vi "_readCmdFromExcel_EEPROM_vna_wmg.vi"(11 "命令类型选择":string(combo)) -> (3 "cmd":string[][](array[string]))   [LabVIEW 2011]
uses:
  <vilib>/Utility/file.llb/Read From Spreadsheet File (string).vi
  <vilib>/Utility/file.llb/Write To Spreadsheet File (string).vi
panel:
  in  "file path (dialog if empty)":path=path "\\\\192.168.20.200\\立讯精密/工程部/电子&测试工程课/临时文件/WMG/HPTS/HPTS_VNA Test System/EEPROM/Commands/Commands1.xls" caption="文件路径 （空时为对话框）"
  out "Loop":i32=5
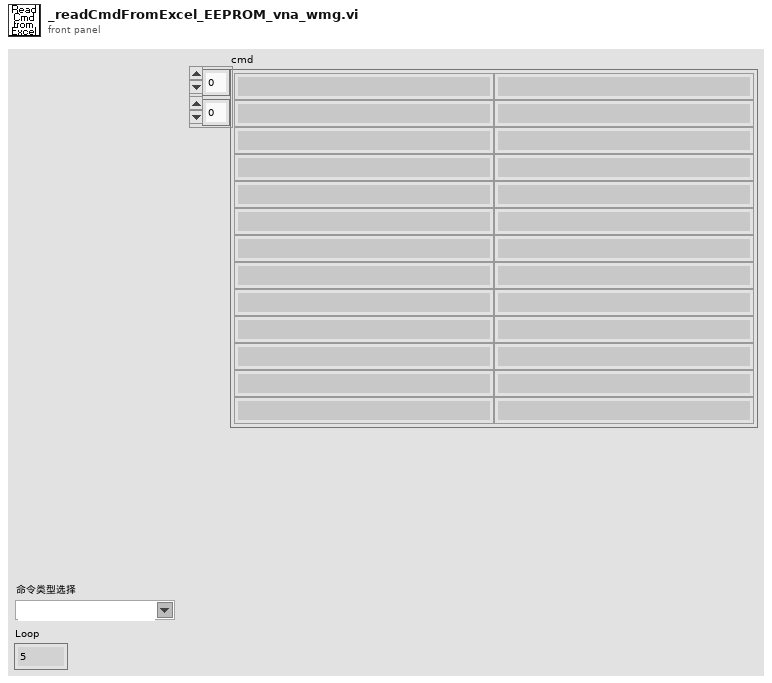
[diagram p1: front panel]
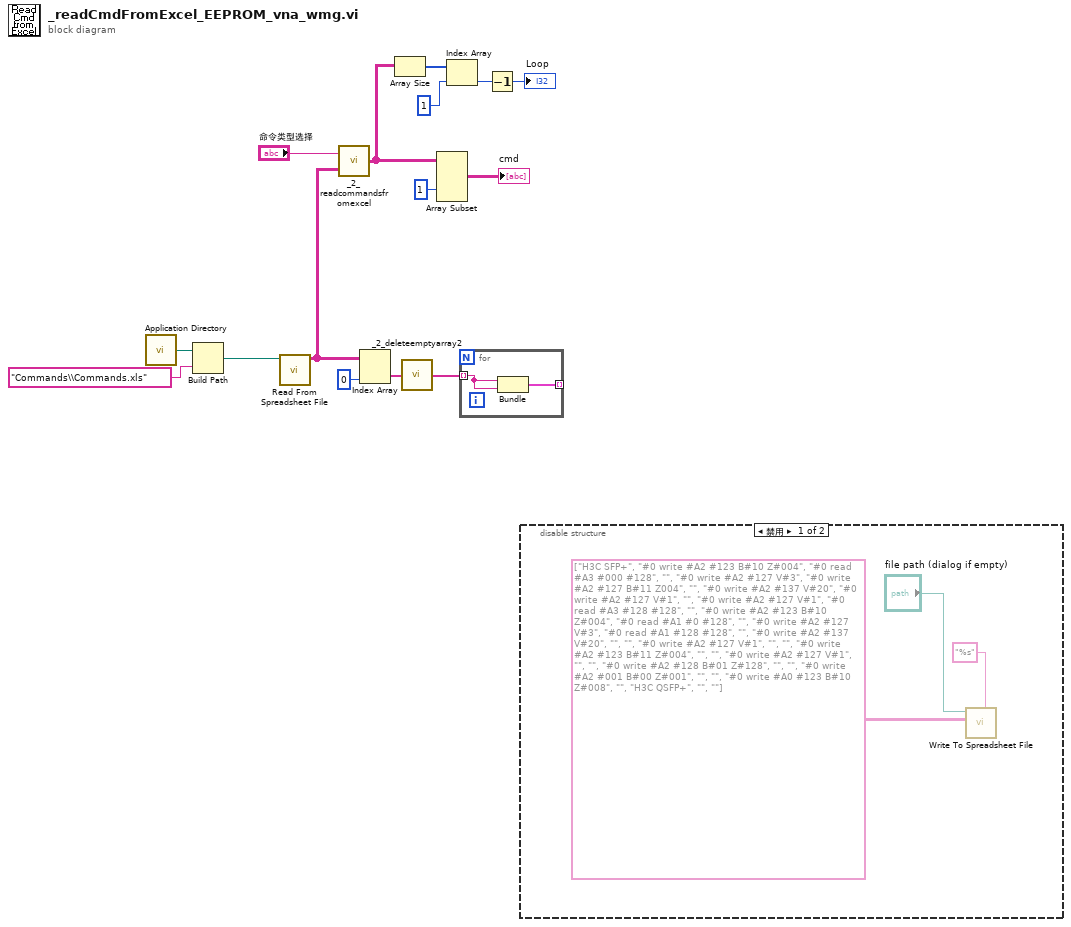
[diagram p0: block diagram]
diagram:
  n1 = call <vilib>:"Application Directory.vi"() -> ("Application Directory"=w15:path)
  n2 = Build Path(base path=w15, name or relative path="Commands\\Commands.xls" ("名称或相对路径")) -> (appended path=w1:path)
  n3 = call-poly <vilib>:"Read From Spreadsheet File.vi"("file path (dialog if empty)"=w1) -> ("all rows"=w4:string[][])  [unwired: 6 in, 4 out]
  n4 = call "_2_readcommandsfromexcel.vi"("inout_chart"=w4, "input_forindex"="命令类型选择") -> ("output"=w9:string[][])
  n5 = Index Array(array=w4, index (col)=0 ("禁用的索引 (列)")) -> (element=w12:string[])  [unwired: 1 in]
  n6 = Array Size(array=w9) -> (size(s)=w6:i32[])
  n7 = call "_2_deleteemptyarray2.vi"("input"=w12) -> ("in_cons"=w11:string[])
  n8 = Array Subset(array=w9, index (col)=1 ("索引")) -> (→"cmd":string[][])  [unwired: 3 in]
  n9 = Index Array(array=w6, index=1 ("索引")) -> (element=w7:i32)
  n10 = for {
    tunnel: w11 -> [w17] mode=indexing
    tunnel: [w16] -> _ mode=indexing
    n11 = Bundle(w17, w17) -> (w16:cluster{string, string})  [unwired: 1 in]
  }
  n12 = Decrement(x=w7) -> (x-1=→"Loop":i32)
  n13 = disable-structure shown="禁用" {
    frame Disabled {
      n14 = call-poly <vilib>:"Write To Spreadsheet File.vi"("format (%s)"="%s", "2D data"=string[][] [["H3C SFP+", "#0 write #A2 #123 B#10 Z#004", "#0 read #A3 #000 #128"], ["", "#0 write #A2 #127 V#3", "#0 write #A2 #127 B#11 Z004"], ["", "#0 write #A2 #137 V#20", "#0 write #A2 #127 V#1"], ["", "#0 write #A2 #127 V#1", "#0 read #A3 #128 #128"], ["", "#0 write #A2 #123 B#10 Z#004", "#0 read #A1 #0 #128"], ["", "#0 write #A2 #127 V#3", "#0 read #A1 #128 #128"], ["", "#0 write #A2 #137 V#20", ""], ["", "#0 write #A2 #127 V#1", ""], ["", "#0 write #A2 #123 B#11 Z#004", ""], ["", "#0 write #A2 #127 V#1", ""], ["", "#0 write #A2 #128 B#01 Z#128", ""], ["", "#0 write #A2 #001 B#00 Z#001", ""], ["", "#0 write #A0 #123 B#10 Z#008", ""], ["H3C QSFP+", "", ""]], "file path (dialog if empty)"="file path (dialog if empty)") -> ()  [unwired: 5 in, 1 out]
    }
    frame Enabled {
    }
  }
